vi "test CRUD device.vi"() -> ()   [LabVIEW 2019]
uses:
  <vilib>/httpClient/POSTBuffer.vi
  <vilib>/httpClient/LabVIEWHTTPClient.lvlib
panel:
  out "id":string
  out "status":string
  out "data":T1(array[cluster])
  out "error out":errorcluster
  out "body":string
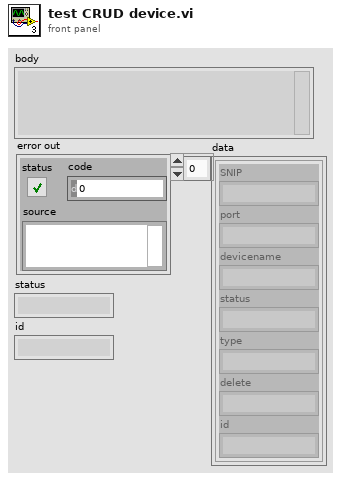
[diagram p1: front panel]
types:
  T1 = cluster{"SNIP":string, "port":string, "devicename":string, "status":string, "type":string, "delete":string, "id":string}[]
  T2 = cluster{"status":string, "data":cluster{"SNIP":string, "port":string, "devicename":string, "status":string, "type":string, "delete":string, "id":string}[]}
  T3 = cluster{"action":string, "SNIP":string, "port":string, "devicename":string, "status":string, "type":string}
  T4 = cluster{"action":string, "SNIP":string, "port":string, "devicename":string, "status":string, "type":string, "id":string}
  T5 = typedef "LabVIEWHTTPClient.lvlib/ClientHandle.ctl" = refnum<k1>
  T6 = cluster{"SNIP":string, "port":string, "devicename":string, "status":string, "type":string, "delete":string, "id":string}
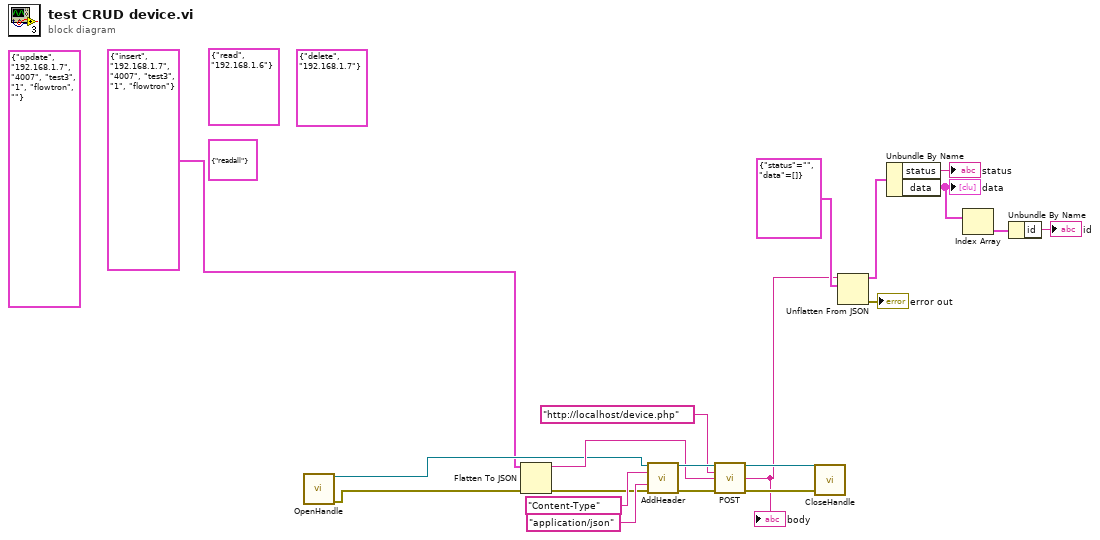
[diagram p0: block diagram]
diagram:
  (unwired) cluster{"action":string} {"action"="readall"}
  (unwired) cluster{"action":string, "SNIP":string} {"action"="delete", "SNIP"="192.168.1.7"}
  (unwired) cluster{"action":string, "SNIP":string} {"action"="read", "SNIP"="192.168.1.6"}
  (unwired) T4 {"action"="update", "SNIP"="192.168.1.7", "port"="4007", "devicename"="test3", "status"="1", "type"="flowtron", "id"=""}
  n1 = call <vilib>:"OpenHandle.vi"() -> ("client handle out"=w11:T5, "error out"=w10:errorcluster)  [unwired: 14 in]
  n2 = Flatten To JSON(anything=T3 {"action"="insert", "SNIP"="192.168.1.7", "port"="4007", "devicename"="test3", "status"="1", "type"="flowtron"}, error in (no error)=w10) -> (JSON string=w15:string, 11:w14:errorcluster)  [unwired: 1 in]
  n3 = call <vilib>:"AddHeader.vi"("client handle"=w11, "header"="Content-Type", "value"="application/json", "error in (no error)"=w14) -> ("client handle out"=w19:T5, "error out"=w20:errorcluster)  [unwired: 10 in]
  n4 = call-poly <vilib>:"POST.vi"("client handle"=w19, "url"="http://localhost/device.php", "buffer"=w15, "error in (no error)"=w20) -> ("client handle out"=w12:T5, "body"=w7:string, "error out"=w13:errorcluster)  [unwired: 8 in, 1 out]
  "body" <- w7
  n5 = call <vilib>:"CloseHandle.vi"("client handle"=w12, "error in (no error)"=w13) -> ()  [unwired: 13 in, 1 out]
  n6 = Unflatten From JSON(JSON string=w7, type and defaults=T2 {"status"="", "data"=[]}) -> (value=w8:T2, error out=→"error out":errorcluster)  [unwired: 5 in]
  n7 = Unbundle By Name(w8) -> ("status"=→"status":string, "data"=w4:T1)
  "data" <- w4
  n8 = Index Array(array=w4) -> (element=w3:T6)  [unwired: 1 in]
  n9 = Unbundle By Name(w3) -> ("id"=→"id":string)
